vi "Write_custom.vi"() -> ()   [LabVIEW 2018]
uses:
  <vilib>/ErrorRing/Error Ring.xnode
panel:
  out "참조 번호 출력":refnum<file>
  out "error out":errorcluster caption="에러 출력"
  in  "error in (no error)":errorcluster caption="에러 입력(에러 없음)"
  in  "정지":bool
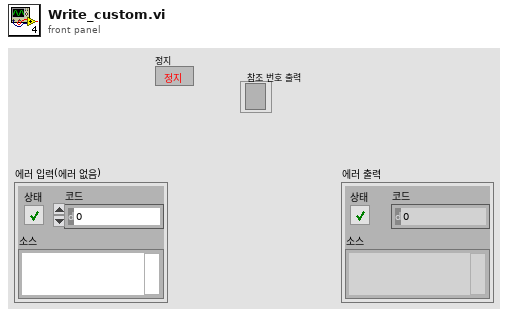
[diagram p1: front panel]
types:
  T1 = enum16{"open", "replace", "create", "open or create", "replace or create", "replace or create with confirmation"}
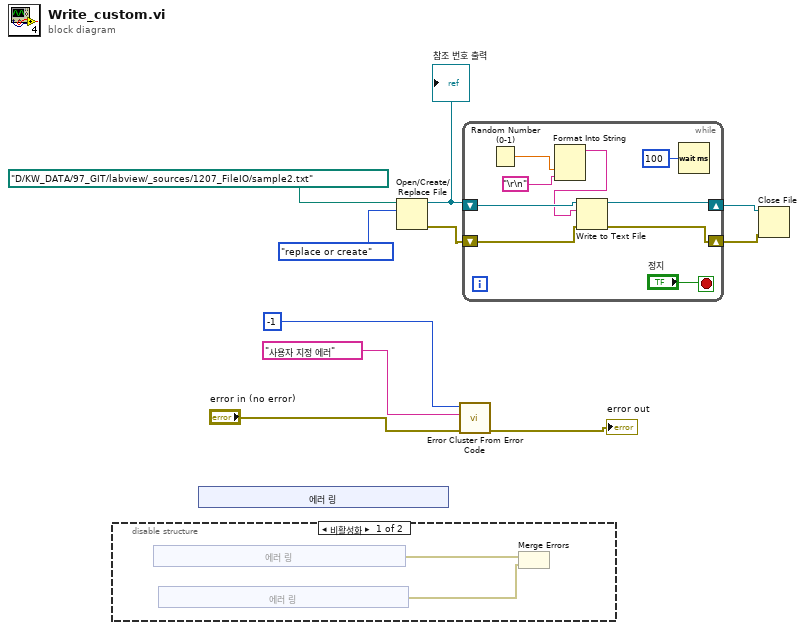
[diagram p0: block diagram]
diagram:
  n1 = disable-structure shown="비활성화" {
    frame Disabled {
      n2 = xnode "에러 링"() -> ("에러 출력"=w12:errorcluster)
      n3 = xnode "에러 링"() -> ("에러 출력"=w11:errorcluster)
      n4 = Merge Errors(w12, w11) -> ()  [unwired: 1 out]
    }
    frame Enabled {
    }
  }
  n5 = xnode "에러 링"() -> ()  [unwired: 1 out]
  n6 = Open/Create/Replace File ("파일 열기/생성/대체")(file path (use dialog)=path "D:/KW_DATA/97_GIT/labview/_sources/1207_FileIO/sample2.txt" ("파일 경로(대화 상자 사용)"), operation (0:open)=T1."replace or create" ("동작(0:open)")) -> (refnum out=w8:refnum<file>, error out=w6:errorcluster)  [unwired: 4 in, 1 out]
  "참조 번호 출력" <- w8
  n7 = call <vilib>:"Error Cluster From Error Code.vi"("error in (no error)"="error in (no error)", "error message (\"\")"="사용자 지정 에러" ("error message (\"\")"), "error code (0)"=-1) -> ("error out"=→"error out":errorcluster)  [unwired: 6 in]
  n8 = while {
    shift-right: [w28] -> w7
    shift-left: w8 -> [w29]
    shift-right: [w26] -> w5
    shift-left: w6 -> [w27]
    stop <- "정지" stop-if-true
    n9 = Random Number (0-1)() -> (number: 0 to 1=w24:dbl)
    n10 = Format Into String(w24, "\r\n") -> (resulting string=w23:string)  [unwired: 3 in, 1 out]
    n11 = Write to Text File(file (use dialog)=w29, text=w23, error in=w27) -> (refnum out=w28:refnum<file>, error out=w26:errorcluster)  [unwired: 1 in, 1 out]
    n12 = Wait (ms)(milliseconds to wait=u32 100 ("대기 시간 (ms)")) -> ()  [unwired: 1 out]
  }
  n13 = Close File(refnum=w7, error in=w5) -> ()  [unwired: 2 out]
